vi "LVFunction_Imop_IsHasoConfigFile.vi"(0 "Configuration file path":path, 11 "error in":errorcluster) -> (4 "IsHasoConfigFile":bool, 15 "error out":errorcluster)   [LabVIEW 2018]
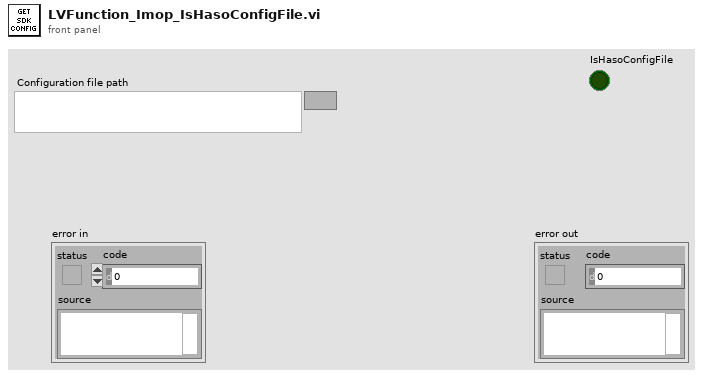
[diagram p1: front panel]
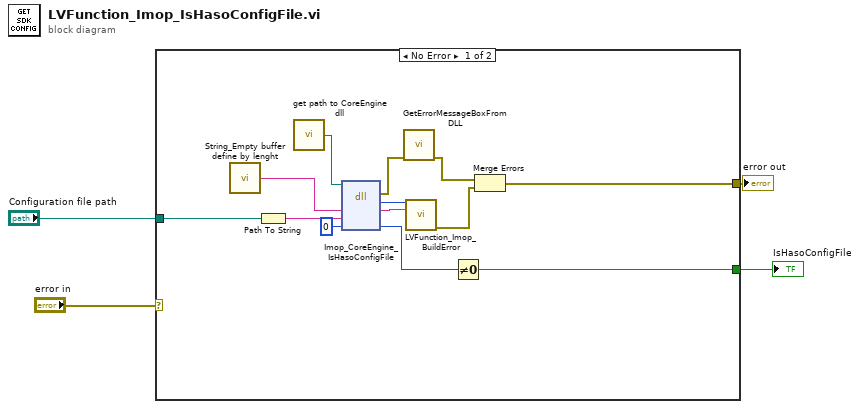
[diagram p0: block diagram]
diagram:
  n1 = case shown="No Error" "error in" {
    selector: "error in" -> [_ w18]
    tunnel: [w10 w18] -> w3
    tunnel: "Configuration file path" -> [w9 _]
    tunnel: [w6 _] -> w1
    frame No Error {
      n2 = call "String_Empty buffer define by lenght.vi"() -> ("Empty buffer"=w11:string)  [unwired: 1 in]
      n3 = Path To String(path=w9) -> (string=w8:string)
      n4 = call "get path to CoreEngine dll.vi"() -> ("path to wavekit library"=w14:path)  [unwired: 14 in, 1 out]
      n5 = dll-call lib="D:/soft/HASO_v3/SVN_trunk/ImOpCoreEngine4_LV2011/DLLs/c_interface_vc100.dll" fn="Imop_CoreEngine_IsHasoConfigFile"(path in=w14, "message"=w11, "config_file_path"=w8, "IsHasoConfigFile"=u8 0) -> (error out=w15:errorcluster, "return type"=w13:i32, "message"=w12:string, "IsHasoConfigFile"=w7:u8)  [unwired: 3 in, 1 out]
      n6 = call "GetErrorMessageBoxFromDLL.vi"("error IN"=w15) -> ("error OUT"=w16:errorcluster)  [unwired: 10 in]
      n7 = call "LVFunction_Imop_BuildError.vi"("code"=w13, "String to Prepend to source (\"\")"=w12) -> ("error out"=w17:errorcluster)  [unwired: 13 in]
      n8 = Not Equal To 0?(x=w7) -> (x != 0?=w6:bool)
      n9 = Merge Errors(w16, w17) -> (w10:errorcluster)
    }
    frame Error {
    }
  }
  "error out" <- w3
  "IsHasoConfigFile" <- w1
